vi "Set Control Input Value.vi"(7 "Vector Component":string, 8 "error in (no error)":errorcluster, 9 "Data":variant, 10 "Control Name":string, 11 "LUnit Test Vector In":refnum<class "LUnit Test Vector.lvclass">) -> (0 "error out":errorcluster, 3 "LUnit Test Vector Out":refnum<class "LUnit Test Vector.lvclass">)   [LabVIEW 2020, in "LUnit Test Vector.lvclass"]
doc: "Sets the control values which will be used when the specified component of the test vector is executed. Front panel controls on the VI under test are referred to by name and must not be on the connector pane of the VI under test."
uses:
  LUnit Test Vector.lvclass
  <vilib>/Utility/miscctls.llb/LVMapReplaceAction.ctl
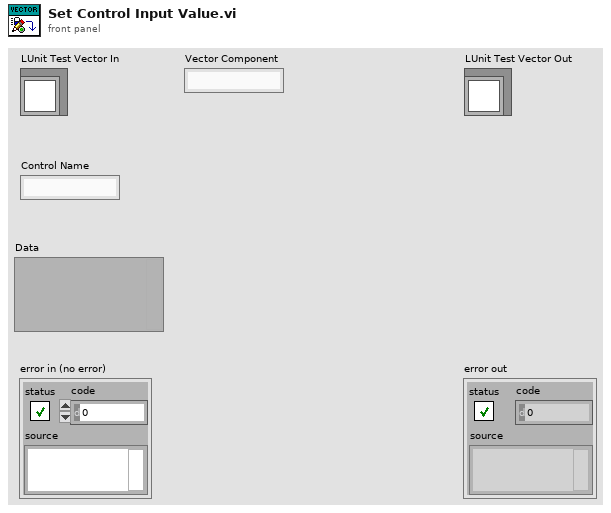
[diagram p1: front panel]
types:
  T1 = typedef "LVMapReplaceAction.ctl" = enum32{"Modify Entry only if found", "Add or Modify Entry", "Delete Entry"}
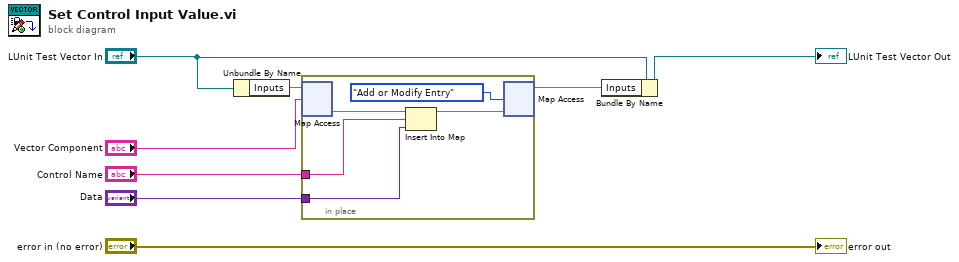
[diagram p0: block diagram]
diagram:
  n1 = Unbundle By Name("LUnit Test Vector In") -> ("Inputs"=w5:map{string, map{string, variant}})
  n2 = in-place {
    in-place-border: "Control Name" -> [w10]
    in-place-border: "Data" -> [w9]
    n3 = in-place-map #1(w5, "Vector Component") -> (w13:map{string, variant})  [unwired: 1 in, 1 out]
    n4 = Insert Into Map(map in=w13, key=w10, value=w9) -> (map out=w12:map{string, variant})  [unwired: 2 out]
    n5 = in-place-map #1(w12, LVMapReplaceAction."Add or Modify Entry" ("action")) -> (w4:map{string, map{string, variant}})  [unwired: 2 out]
  }
  n6 = Bundle By Name(cluster="LUnit Test Vector In", "Inputs"=w4) -> (→"LUnit Test Vector Out":refnum<class "LUnit Test Vector.lvclass">)
  "error out" <- "error in (no error)"
